vi "create2.vi"(6 "actual y size":i32, 9 "center":i32, 10 "X size":i32, 11 "max Y size":i32) -> (2 "size":i32, 3 "Array":i32[][](array[numeric]))   [LabVIEW 2013]
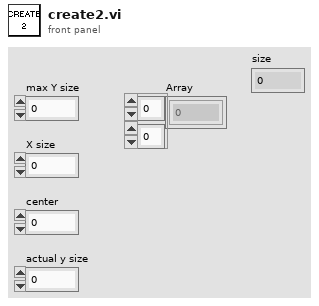
[diagram p1: front panel]
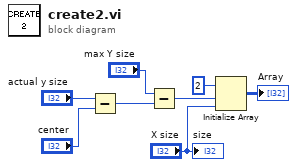
[diagram p0: block diagram]
diagram:
  n1 = Subtract(x="actual y size", y="center") -> (x-y=w5:i32)
  n2 = Subtract(x="max Y size", y=w5) -> (x-y=w3:i32)
  n3 = Initialize Array(2, w3, "X size") -> (→"Array":i32[][])
  "size" <- "X size"
